vi "H036 Harsh Pandit SCADA Lab 9 Sem 6.vi"() -> ()   [LabVIEW 2018]
uses:
  <vilib>/LabVIEW Interface for Arduino/Type Defs/Board Type.ctl
  <vilib>/LabVIEW Interface for Arduino/Type Defs/Pin Mode.ctl
  <vilib>/LabVIEW Interface for Arduino/LabVIEW Interface for Arduino.lvlib
panel:
  in  "Pin Mode (Input)":T1
  in  "Boolean":bool
  in  "Board Type (Uno)":T2
  in  "VISA resource":refnum<visa-resource-name>
  # "Experiment 9 : Develope a HMI to switch on an off inbuilt LED at pin 13 of \nArduino."
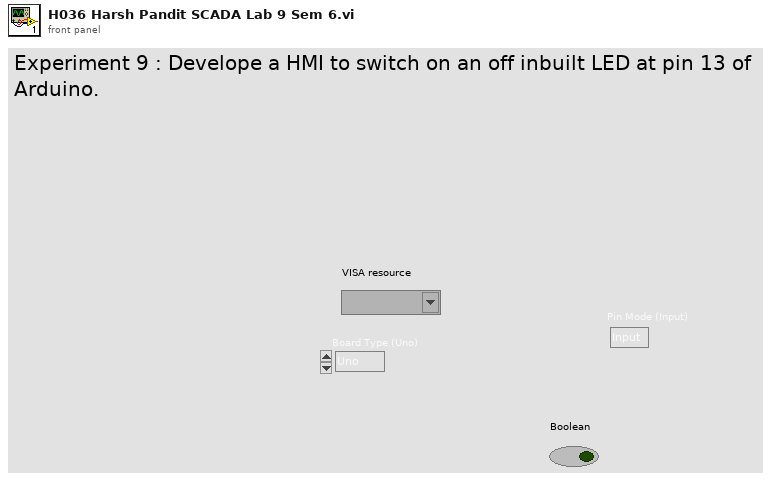
[diagram p1: front panel]
types:
  T1 = typedef "LabVIEW Interface for Arduino.lvlib/Pin Mode.ctl" = enum8{"Input", "Output"}
  T2 = typedef "LabVIEW Interface for Arduino.lvlib/Board Type.ctl" = enum16{"Uno", "Dimuelanove w/Atmega 328", "Mega 2560"}
  T3 = typedef "LabVIEW Interface for Arduino.lvlib/Arduino Resource.ctl" = cluster{"VISA resource":refnum<visa-resource-name>, "Board Type":T2, "Connection Type":enum8{"USB / Serial"}, "Bytes Per Packet (15)":u8}
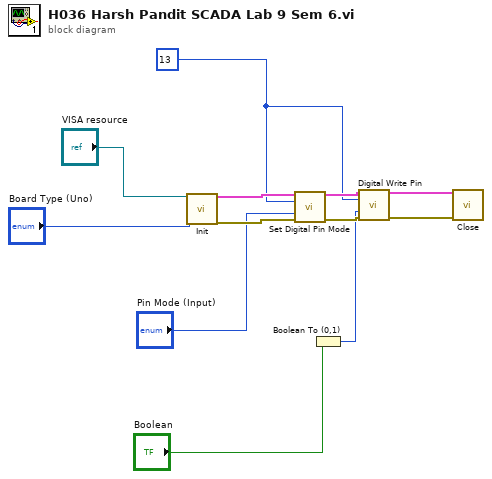
[diagram p0: block diagram]
diagram:
  w1 = u8 13 ("Digital I/O Pin")
  n1 = call <vilib>:"Init.vi"("VISA resource"="VISA resource", "Board Type (Uno)"="Board Type (Uno)") -> ("Arduino Resource"=w10:T3, "error out"=w9:errorcluster)  [unwired: 16 in]
  n2 = call <vilib>:"Set Digital Pin Mode.vi"("Arduino Resource"=w10, "Digital I/O Pin"=w1, "Pin Mode (Input)"="Pin Mode (Input)", "error in"=w9) -> ("Arduino Resource"=w8:T3, "error out"=w7:errorcluster)  [unwired: 10 in]
  n3 = Boolean To (0,1)(Boolean="Boolean") -> (0, 1=w6:i16)
  n4 = call <vilib>:"Digital Write Pin.vi"("Arduino Resource"=w8, "Digital I/O Pin (0)"=w1, "Value (0)"=w6, "error in"=w7) -> ("Arduino Resource"=w5:T3, "error out"=w4:errorcluster)  [unwired: 10 in]
  n5 = call <vilib>:"Close.vi"("Arduino Resource"=w5, "error in"=w4) -> ()  [unwired: 13 in, 1 out]
